vi "Main.vi"() -> ()   [LabVIEW 2018]
uses:
  <vilib>/MakerHub/LINX/Private/Type Defs/Interface.ctl
  <vilib>/MakerHub/LINX/Public/Initialize.vi
  <vilib>/MakerHub/LINX/Public/Sensors/Motion/Servo/Servo Open One Channel.vi
  <vilib>/MakerHub/LINX/LMH-LINX.lvlib
  <vilib>/MakerHub/LINX/Public/Sensors/Motion/Servo/Servo.lvlib
panel:
  out "Waveform Chart":dbl(graph)
  in  "Error In":errorcluster
  in  "MANUAL PUMP SET":bool
  out "Modality":enum8{"Manuale", "Automatico"}(ring)
  in  "stop":bool
  out "error out":errorcluster
  in  "Modalità":bool
  in  "Serial port":refnum<visa-resource-name>
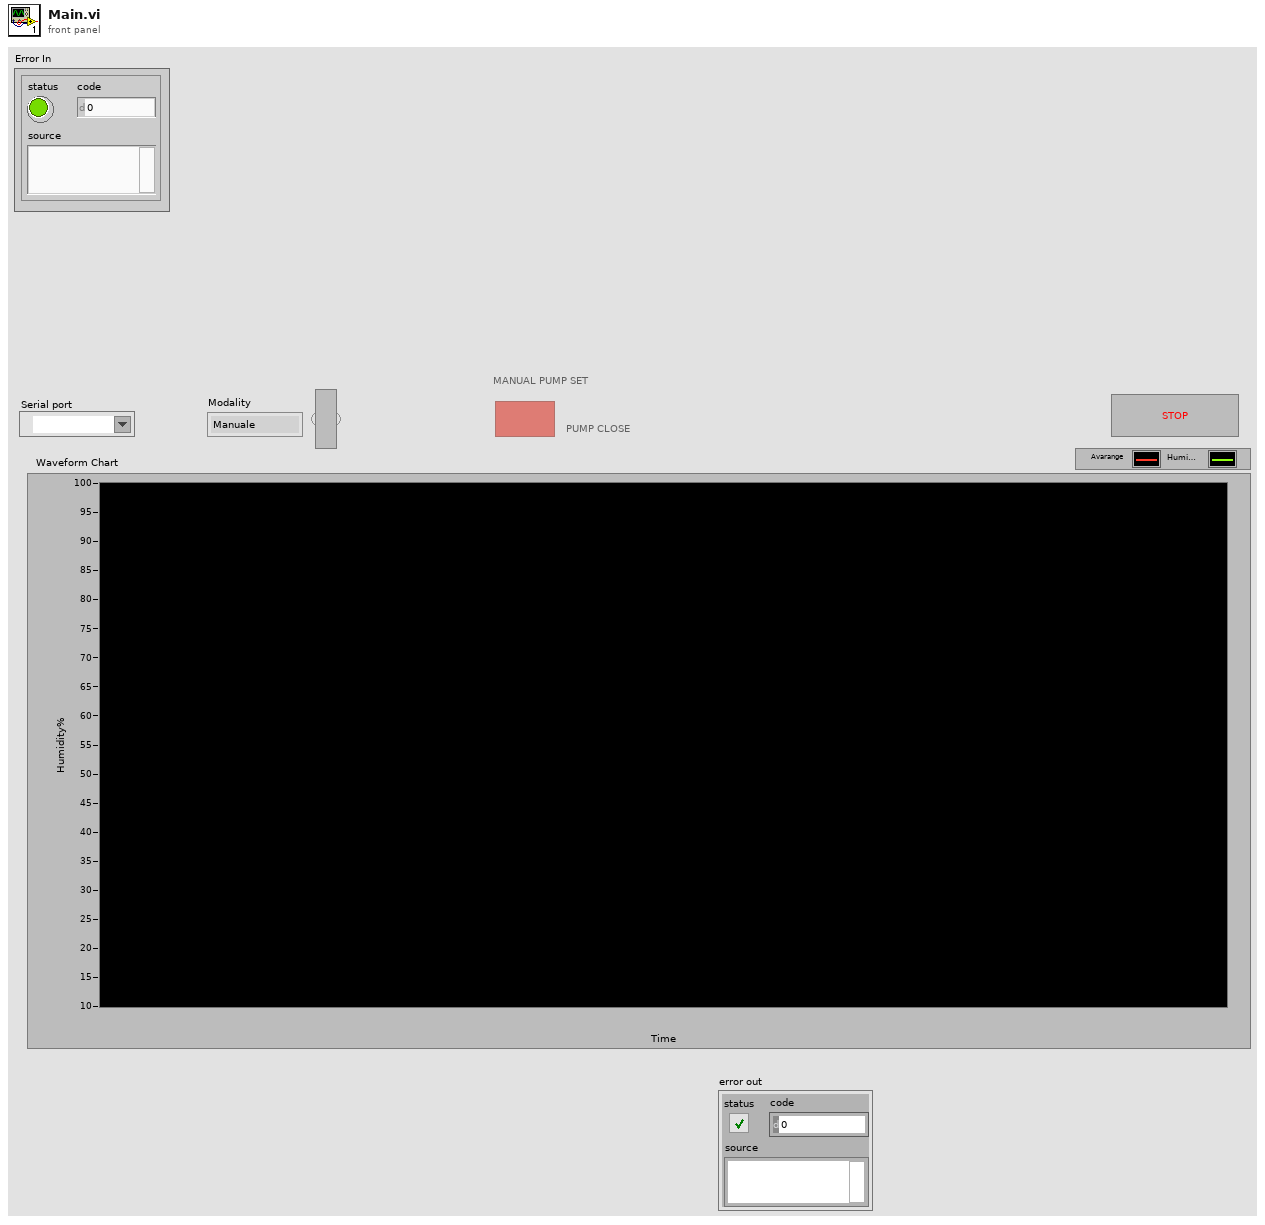
[diagram p1: front panel]
types:
  T1 = typedef "LMH-LINX.lvlib/Interface.ctl" = enum16{"Serial", "TCP"}
  T2 = typedef "LMH-LINX.lvlib/LINX Ref.ctl" = cluster{"IO":T3, "Interface":T1, "LINX Device Config":T4}
  T3 = typedef "LMH-LINX.lvlib/Platform.ctl" = enum16{"Remote", "Local"}
  T4 = typedef "LMH-LINX.lvlib/Device.lvlib/LINX Device Config.ctl" = cluster{"Interface":T1, "COM Port":refnum<visa-resource-name>, "TCP Configuration":T5, "Device Family":u8, "Device ID":u8, "Device Name":string, "TCP Ref":refnum<k5>, "Channels":T6}
  T5 = typedef "LMH-LINX.lvlib/Device.lvlib/TCP Config.ctl" = cluster{"IP Address":string, "Port":u16}
  T6 = typedef "LMH-LINX.lvlib/Channels.ctl" = cluster{"DI":u8[], "DO":u8[], "AI":u8[], "AO":u8[], "PWM":u8[], "QE":u8[], "UART":u8[], "I2C 2":u8[], "SPI":u8[], "CAN":u8[], "Servo":u8[], "AI Ref (V)":dbl, "AI Resolution (Bits)":u8, "AO Ref (V)":dbl, "AO Resolution (Bits)":u8}
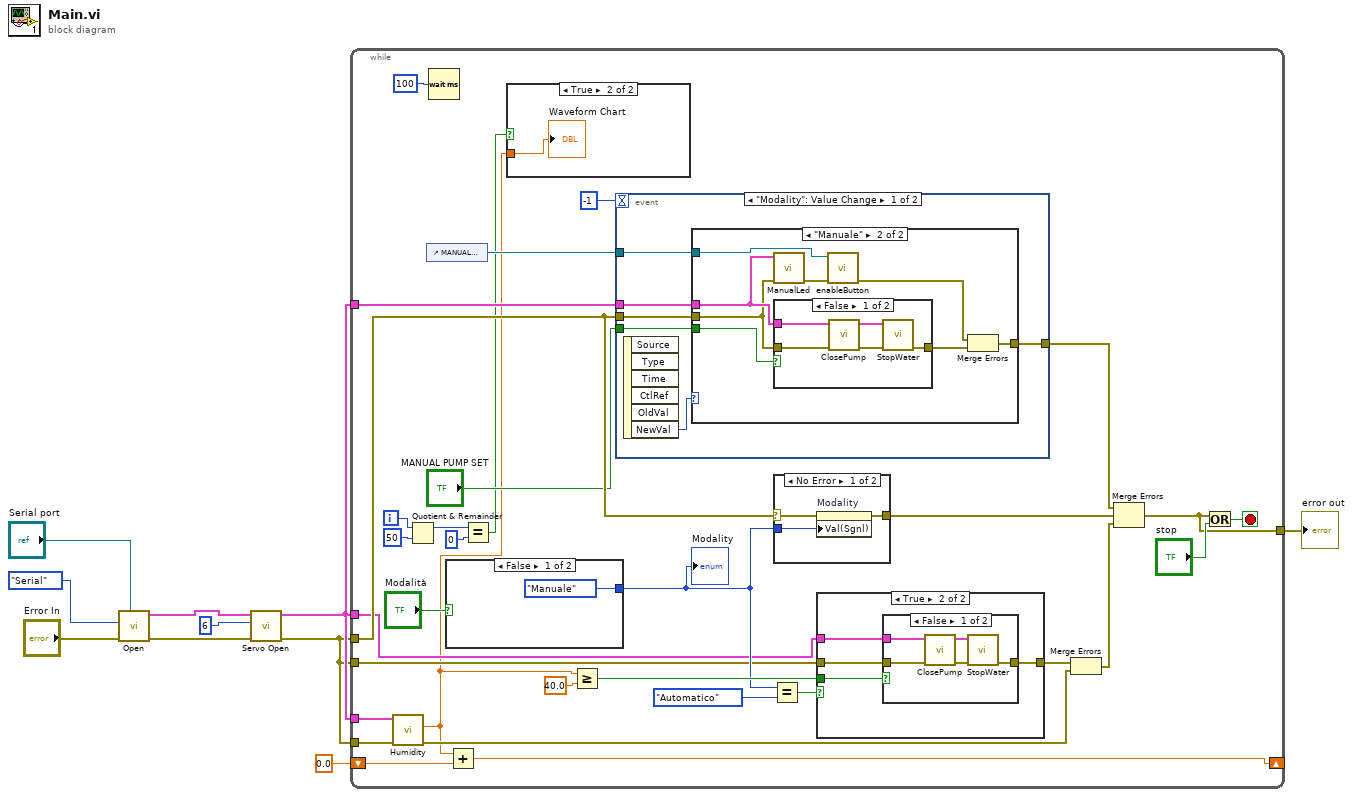
[diagram p0: block diagram]
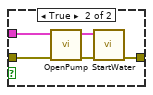
[diagram p4: hidden frame]
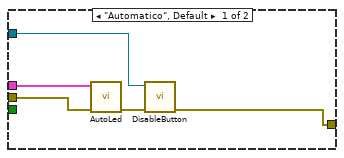
[diagram p6: hidden frame]
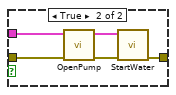
[diagram p7: hidden frame]
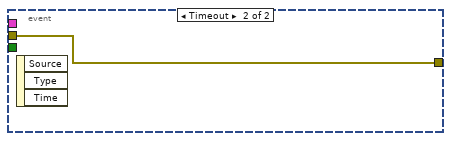
[diagram p8: hidden frame]
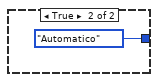
[diagram p9: hidden frame]
diagram:
  n1 = call-poly <vilib>:"Open.vi"("Serial Port"="Serial port", "Error In"="Error In", "Interface"=Interface."Serial") -> ("Error Out"=w5:errorcluster, "LINX Resource"=w1:T2)  [unwired: 6 in, 1 out]
  n2 = call-poly <vilib>:"Servo Open.vi"("Error In"=w5, "Servo Channel"=u8 6, "LINX Resource"=w1) -> ("Error Out"=w2:errorcluster, "LINX Resource"=w3:T2)  [unwired: 7 in]
  n3 = while {
    tunnel: w2 -> [w30]
    tunnel: w3 -> [w27]
    tunnel: w3 -> [w37]
    shift-right: [w21] -> _
    shift-left: 0.0 ("Humidity") -> [w12]
    tunnel: [w29] -> w8
    tunnel: w2 -> [w24]
    tunnel: w2 -> [w17]
    tunnel: w3 -> [w16]
    i -> [w19]
    stop <- w32 stop-if-true
    n4 = call "Humidity.vi"("error in (no error)"=w24, "LINX Resource in"=w27) -> ("error out"=w15:errorcluster, "Humidity"=w11:dbl)  [unwired: 8 in]
    n5 = Quotient & Remainder(x=w19, y=50) -> (x-y*floor(x/y)=w20:i32)  [unwired: 1 out]
    n6 = control-ref of="MANUAL PUMP SET"() -> (w28:refnum<vi>)
    n7 = Wait (ms)(milliseconds to wait=u32 100 ("millisecond timer value")) -> ()  [unwired: 1 out]
    n8 = case shown="False" "Modalità" {
      tunnel: [enum8{"Manuale", "Automatico"}."Manuale" ("Modality") enum8{"Manuale", "Automatico"}."Automatico" ("Modality")] -> w22
      frame False {
      }
      frame True {
      }
    }
    "Modality" <- w22
    n9 = Add(x=w11, y=w12) -> (x+y=w21:dbl)
    n10 = Equal?(x=w20, y=0) -> (x = y?=w18:bool)
    n11 = case shown="True" w18 {
      tunnel: w11 -> [_ w43]
      frame False {
      }
      frame True {
        "Waveform Chart" <- w43
      }
    }
    n12 = Greater Or Equal?(x=w11, y=40.0) -> (x >= y?=w34:bool)
    n13 = event shown="[0] \"Modality\": Value Change" {
      selector: _ -> [_ _]
      dyn-events: _ -> [_ _]
      timeout: -1 -> [_ _]
      tunnel: w30 -> [w66 w92]
      tunnel: w37 -> [w67 _]
      tunnel: [w65 w92] -> w25
      tunnel: w28 -> [w64 _]
      tunnel: "MANUAL PUMP SET" -> [w63 _]
      event "Modality": Value Change {
        n14 = event-data() -> ("NewVal"=w68:enum8{"Manuale", "Automatico"})  [unwired: 1 in, 5 out]
        n15 = case shown="\"Manuale\"" w68 {
          tunnel: w67 -> [w69 w78]
          tunnel: w66 -> [w73 w77]
          tunnel: [w71 w74] -> w65
          tunnel: w64 -> [w70 w80]
          tunnel: w63 -> [_ w79]
          frame "Automatico", Default {
            n16 = call "AutoLed.vi"("error in (no error)"=w73, "LINX Resource"=w69) -> ("error out"=w72:errorcluster)  [unwired: 9 in]
            n17 = call "DisableButton.vi"("error in (no error)"=w72, "Boolean in"=w70) -> ("error out"=w71:errorcluster)  [unwired: 9 in]
          }
          frame "Manuale" {
            n18 = call "ManualLed.vi"("error in (no error)"=w77, "LINX Resource"=w78) -> ("error out"=w81:errorcluster)  [unwired: 9 in]
            n19 = case shown="False" w79 {
              tunnel: w78 -> [w85 w91]
              tunnel: w77 -> [w84 w90]
              tunnel: [w86 w87] -> w76
              frame False {
                n20 = call "ClosePump.vi"("error in (no error)"=w84, "LINX Resource in"=w85) -> ("error out"=w83:errorcluster, "LINX Resource"=w82:T2)  [unwired: 8 in]
                n21 = call "StopWater.vi"("error in (no error)"=w83, "LINX Resource in"=w82) -> ("error out"=w86:errorcluster)  [unwired: 8 in, 1 out]
              }
              frame True {
                n22 = call "OpenPump.vi"("error in (no error)"=w90, "LINX Resource in"=w91) -> ("error out"=w88:errorcluster, "LINX Resource"=w89:T2)  [unwired: 8 in]
                n23 = call "StartWater.vi"("error in (no error)"=w88, "LINX Resource in"=w89) -> ("error out"=w87:errorcluster)  [unwired: 8 in, 1 out]
              }
            }
            n24 = call "enableButton.vi"("error in (no error)"=w81, "Boolean in"=w80) -> ("error out"=w75:errorcluster)  [unwired: 9 in]
            n25 = Merge Errors(w75, w76) -> (w74:errorcluster)
          }
        }
      }
      event Timeout {
        n26 = event-data() -> ()  [unwired: 1 in, 3 out]
      }
    }
    n27 = Equal?(x=w22, y=enum8{"Manuale", "Automatico"}."Automatico") -> (x = y?=w35:bool)
    n28 = case shown="No Error" w30 {
      selector: w30 -> [w60 w62]
      tunnel: w22 -> [w61 _]
      tunnel: [w59 w62] -> w40
      frame No Error {
        n29 = property on="Modality" class="Enum (strict)"(error in=w60, "Val(Sgnl)"=w61) -> (error out=w59:errorcluster)  [unwired: 1 in, 1 out]
      }
      frame Error {
      }
    }
    n30 = case shown="True" w35 {
      tunnel: w34 -> [_ w48]
      tunnel: w16 -> [_ w47]
      tunnel: w17 -> [w44 w46]
      tunnel: [w44 w45] -> w14
      frame False {
      }
      frame True {
        n31 = case shown="False" w48 {
          tunnel: w46 -> [w53 w57]
          tunnel: w47 -> [w52 w58]
          tunnel: [w49 w54] -> w45
          frame False {
            n32 = call "ClosePump.vi"("error in (no error)"=w53, "LINX Resource in"=w52) -> ("error out"=w50:errorcluster, "LINX Resource"=w51:T2)  [unwired: 8 in]
            n33 = call "StopWater.vi"("error in (no error)"=w50, "LINX Resource in"=w51) -> ("error out"=w49:errorcluster)  [unwired: 8 in, 1 out]
          }
          frame True {
            n34 = call "OpenPump.vi"("error in (no error)"=w57, "LINX Resource in"=w58) -> ("error out"=w56:errorcluster, "LINX Resource"=w55:T2)  [unwired: 8 in]
            n35 = call "StartWater.vi"("error in (no error)"=w56, "LINX Resource in"=w55) -> ("error out"=w54:errorcluster)  [unwired: 8 in, 1 out]
          }
        }
      }
    }
    n36 = Merge Errors(w14, w15) -> (w13:errorcluster)
    n37 = Merge Errors(w25, w40, w13) -> (w29:errorcluster)
    n38 = Or(x=w29, y="stop") -> (x .or. y?=w32:bool)
  }
  "error out" <- w8
